vi "天数计算.vi"(10 "天数":dbl) -> (0 "error constant":errorcluster, 1 "月份":string, 3 "日期":string)   [LabVIEW 2011]
panel:
  out "年份":string
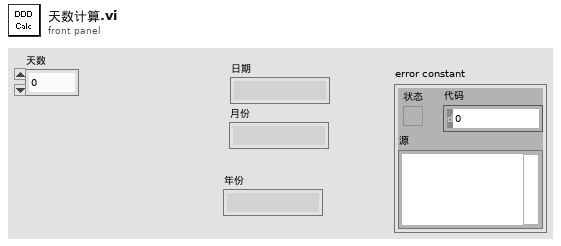
[diagram p1: front panel]
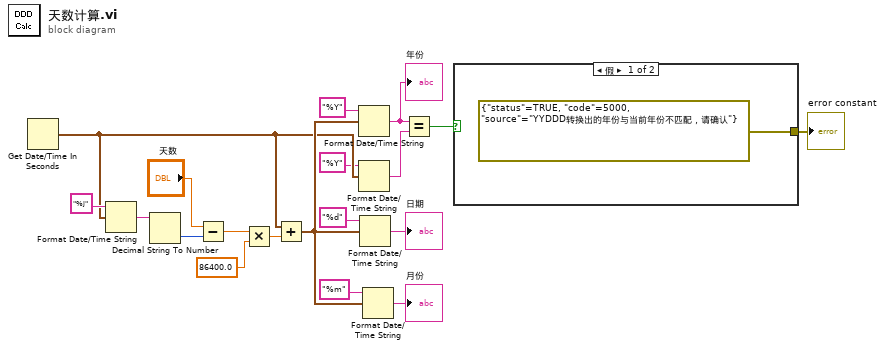
[diagram p0: block diagram]
diagram:
  n1 = Get Date/Time In Seconds() -> (seconds since 1Jan1904=w6:timestamp)
  n2 = Format Date/Time String(time format string (%c)="%j" ("时间格式字符串(%c)"), seconds (now)=w6) -> (date/time string=w18:string)  [unwired: 1 in]
  n3 = Decimal String To Number(string=w18) -> (number=w12:i32)  [unwired: 2 in, 1 out]
  n4 = Subtract(x="天数", y=w12) -> (x-y=w17:dbl)
  n5 = Multiply(x=w17, y=86400.0) -> (x*y=w15:dbl)
  n6 = Add(x=w6, y=w15) -> (x+y=w8:timestamp)
  n7 = Format Date/Time String(time format string (%c)="%Y" ("时间格式字符串(%c)"), seconds (now)=w8) -> (date/time string=w4:string)  [unwired: 1 in]
  "年份" <- w4
  n8 = Format Date/Time String(time format string (%c)="%Y" ("时间格式字符串(%c)"), seconds (now)=w6) -> (date/time string=w3:string)  [unwired: 1 in]
  n9 = Format Date/Time String(time format string (%c)="%d" ("时间格式字符串(%c)"), seconds (now)=w8) -> (date/time string=→"日期":string)  [unwired: 1 in]
  n10 = Format Date/Time String(time format string (%c)="%m" ("时间格式字符串(%c)"), seconds (now)=w8) -> (date/time string=→"月份":string)  [unwired: 1 in]
  n11 = Equal?(x=w4, y=w3) -> (x = y?=w2:bool)
  n12 = case shown="假" w2 {
    tunnel: [errorcluster {"status"=TRUE, "code"=5000, "source"="YYDDD转换出的年份与当前年份不匹配，请确认"} ("error constant") _] -> w1
    frame False {
    }
    frame True {
    }
  }
  "error constant" <- w1
